vi "CarWash_1-Panel.vi"() -> ()   [LabVIEW 2021]
uses:
  Global-Var-Simulator.vi
  Global-Var-ControlPanel.vi
panel:
  in  "delete_all_alarams":bool
  out "broken_nozzle":bool
  out "high_temp":bool
  out "high_press":bool
  out "pump_clogged":bool
  out "shiner_low_level":bool
  out "soap_low_level":bool
  out "water_low_level":bool
  out "shiner_level_ind":dbl
  out "soap_level_ind":dbl
  out "water_level_ind":dbl
  out "shiner_level_tank":dbl(slide) scale=0.0..500.0
  out "soap_level_tank":dbl(slide) scale=0.0..500.0
  out "water_level_tank":dbl(slide) scale=0.0..500.0
  in  "home_btn":bool
  # "Myjnia Południe"
  # "Niski poziom wody"
  # "Niski poziom mydła"
  # "Poziomy płynów w zbiornikach"
  # "Niski poziom nabłyszczacza"
  # "Woda"
  # "Mydło"
  # "Nabłyszczacz"
  # "Zatkana pompa"
  # "Wysokie ciśnienie"
  # "Wysoka temperatura"
  # "Złamana dysza"
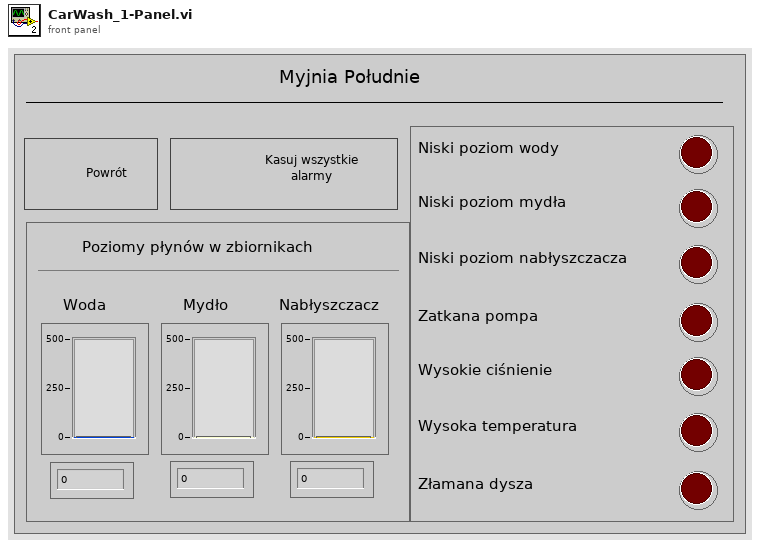
[diagram p1: front panel]
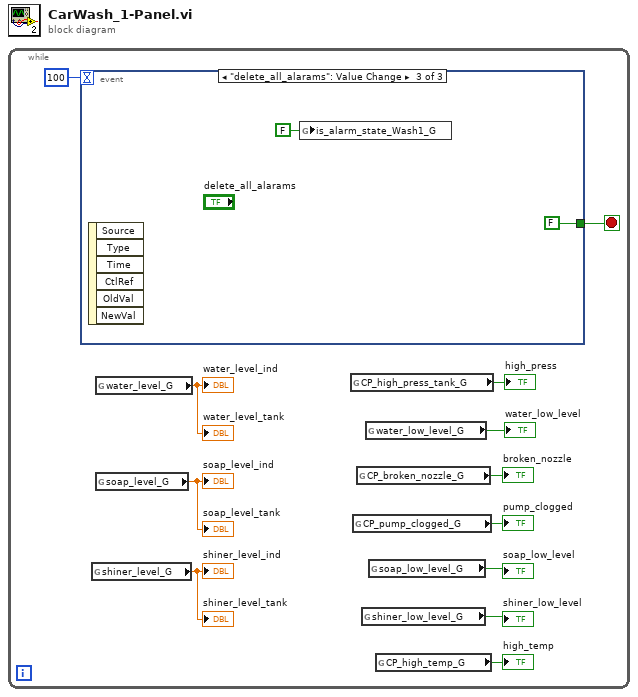
[diagram p0: block diagram]
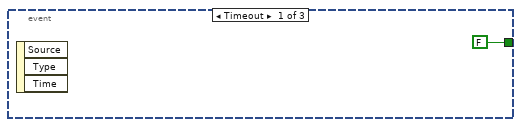
[diagram p2: hidden frame]
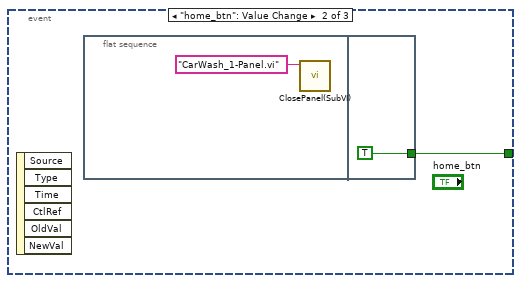
[diagram p3: hidden frame]
diagram:
  n1 = while {
    stop <- w12 stop-if-true
    n2 = event shown="[2] \"delete_all_alarams\": Value Change" {
      selector: _ -> [_ _ _]
      dyn-events: _ -> [_ _ _]
      timeout: 100 -> [_ _ _]
      tunnel: [FALSE w14 FALSE] -> w12
      event Timeout {
        n3 = event-data() -> ()  [unwired: 1 in, 3 out]
      }
      event "home_btn": Value Change {
        n4 = event-data() -> ()  [unwired: 1 in, 6 out]
        n5 = flat-sequence {
          tunnel: [TRUE] -> w14
          frame #0 {
            n6 = call "ClosePanel(SubVI).vi"("String"="CarWash_1-Panel.vi") -> ()  [unwired: 11 in]
          }
          frame #1 {
          }
        }
      }
      event "delete_all_alarams": Value Change {
        n7 = event-data() -> ()  [unwired: 1 in, 6 out]
        n8 = global write "Global-Var-Simulator.vi" "is_alarm_state_Wash1_G"(FALSE ("is_alarm_state_Wash1_G")) -> ()
      }
    }
    n9 = global read "Global-Var-Simulator.vi" "shiner_level_G"() -> (→"shiner_level_tank" →"shiner_level_ind":dbl)
    n10 = global read "Global-Var-Simulator.vi" "water_level_G"() -> (→"water_level_tank" →"water_level_ind":dbl)
    n11 = global read "Global-Var-Simulator.vi" "soap_level_G"() -> (→"soap_level_tank" →"soap_level_ind":dbl)
    n12 = global read "Global-Var-ControlPanel.vi" "CP_high_press_tank_G"() -> (→"high_press":bool)
    n13 = global read "Global-Var-ControlPanel.vi" "CP_pump_clogged_G"() -> (→"pump_clogged":bool)
    n14 = global read "Global-Var-ControlPanel.vi" "CP_broken_nozzle_G"() -> (→"broken_nozzle":bool)
    n15 = global read "Global-Var-Simulator.vi" "shiner_low_level_G"() -> (→"shiner_low_level":bool)
    n16 = global read "Global-Var-Simulator.vi" "water_low_level_G"() -> (→"water_low_level":bool)
    n17 = global read "Global-Var-Simulator.vi" "soap_low_level_G"() -> (→"soap_low_level":bool)
    n18 = global read "Global-Var-ControlPanel.vi" "CP_high_temp_G"() -> (→"high_temp":bool)
  }
